vi "Write Values.vi"(10 "Values":variant[][](array[variant]), 11 "Series in":refnum<class "Series.lvclass">) -> (3 "Series out":refnum<class "Series.lvclass">)   [LabVIEW 2017]
uses:
  Series.lvclass
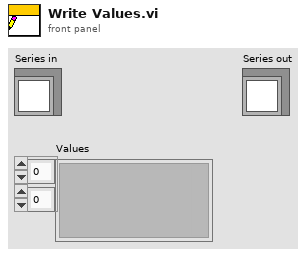
[diagram p1: front panel]
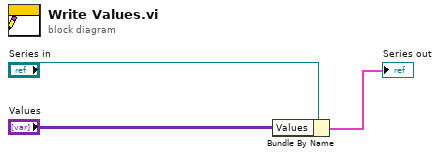
[diagram p0: block diagram]
diagram:
  n1 = Bundle By Name(cluster="Series in", "Values"="Values") -> (→"Series out":cluster{})
